vi "LWXPS_TimerGet.vi"(0 "XPS Reference IN":refnum<k24>, 7 "Timer Name":string, 11 "LabVIEW error IN":errorcluster) -> (4 "XPS Reference OUT":refnum<k24>, 6 "Returned error code":i32, 8 "Frequency Ticks":i32, 10 "XPS Error String":string, 15 "LabVIEW error OUT":errorcluster)   [LabVIEW 2014]
uses:
  D:/XPSQ8_LabView_Library/Development/Source/Dll/Newport.XPS.CommandInterface.dll
  Dll/Newport.XPS.CommandInterface.dll
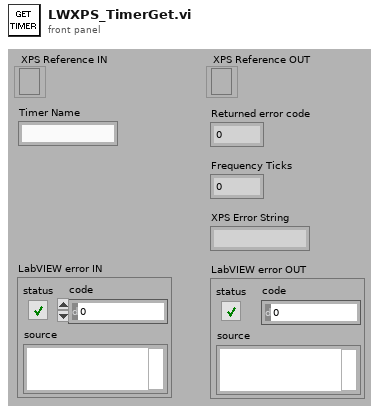
[diagram p1: front panel]
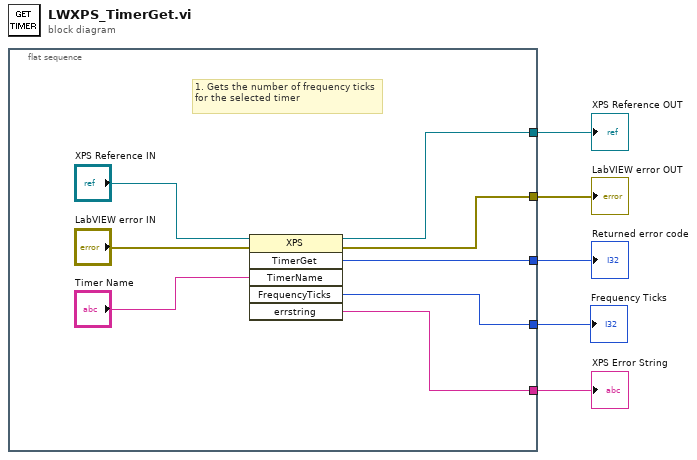
[diagram p0: block diagram]
diagram:
  n1 = flat-sequence {
    tunnel: [w11] -> w5
    tunnel: [w8] -> w4
    tunnel: [w12] -> w3
    tunnel: [w6] -> w1
    tunnel: [w7] -> w2
    frame #0 {
      # "1. Gets the number of frequency ticks for the selected timer"
      n2 = invoke class="XPS" method="TimerGet"(reference="XPS Reference IN", error in="LabVIEW error IN", "TimerName"="Timer Name") -> (reference out=w11:refnum<k24>, error out=w8:errorcluster, "TimerGet"=w12:i32, "FrequencyTicks"=w6:i32, "errstring"=w7:string)  [unwired: 3 in, 1 out]
    }
  }
  "XPS Error String" <- w2
  "XPS Reference OUT" <- w5
  "LabVIEW error OUT" <- w4
  "Returned error code" <- w3
  "Frequency Ticks" <- w1
